vi "12.14.15 Voltage input8inputs.vi"(0 "refnum Write file in":refnum<file>, 1 "Stop in":refnum<vi>, 3 "Number of Samples":i32=100, 4 "Sample Rate":dbl=1000.0, 7 "error in 2":errorcluster, 8 "Display? \nOff/On":bool, 10 "Boolean":bool, 11 "Sample rate (actual)":refnum<vi>, 15 "Plot Output":refnum<vi>, 16 "Plot 1 ref":refnum<vi>, 17 "Plot 2 ref":refnum<vi>) -> (13 "error out 2":errorcluster, 14 "refnum Write file out":refnum<file>, 19 "error out":errorcluster)   [LabVIEW 2017]
uses:
  <vilib>/DAQmx/read.llb/DAQmx Read (Analog 1D Wfm NChan NSamp).vi
  <vilib>/DAQmx/create/channels.llb/DAQmx Create Channel (AI-Voltage-Basic).vi
  <vilib>/DAQmx/configure/timing.llb/DAQmx Timing (Sample Clock).vi
  <vilib>/DAQmx/miscellaneous.llb/DAQmx Fill In Error Info.vi
  <resource>/objmgr/daqmx.rc
panel:
  out "Plot 3":cluster{dbl, dbl, dbl, dbl}(graph)
  out "Plot 1":dbl(graph)
  out "Plot 2":dbl(graph)
  out "Actual Sample Rate":dbl=1000.0 format="%0.2f"
  # "© The Regents of the University of California, Davis campus, 2019. This material is available as open source for research and personal use under a Creative Commons Attribution-NonCommercial-NoDerivatives 4.0 International Public License (https://creativecommons.org/licenses/by-nc-nd/4.0/)."
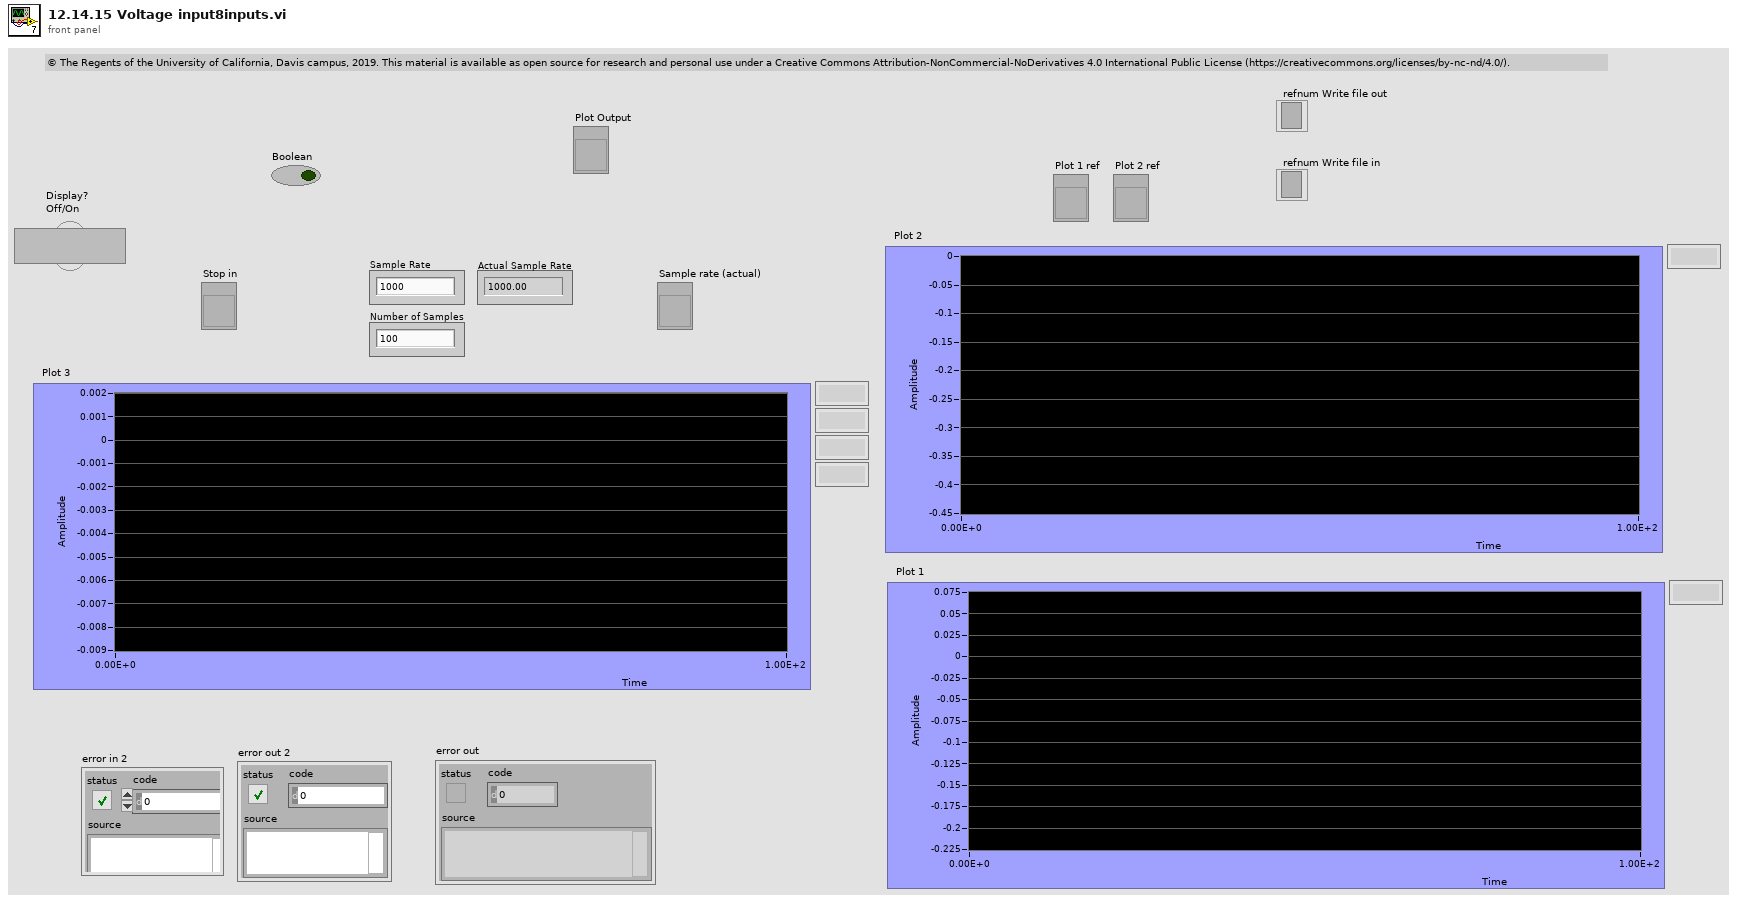
[diagram p1: front panel]
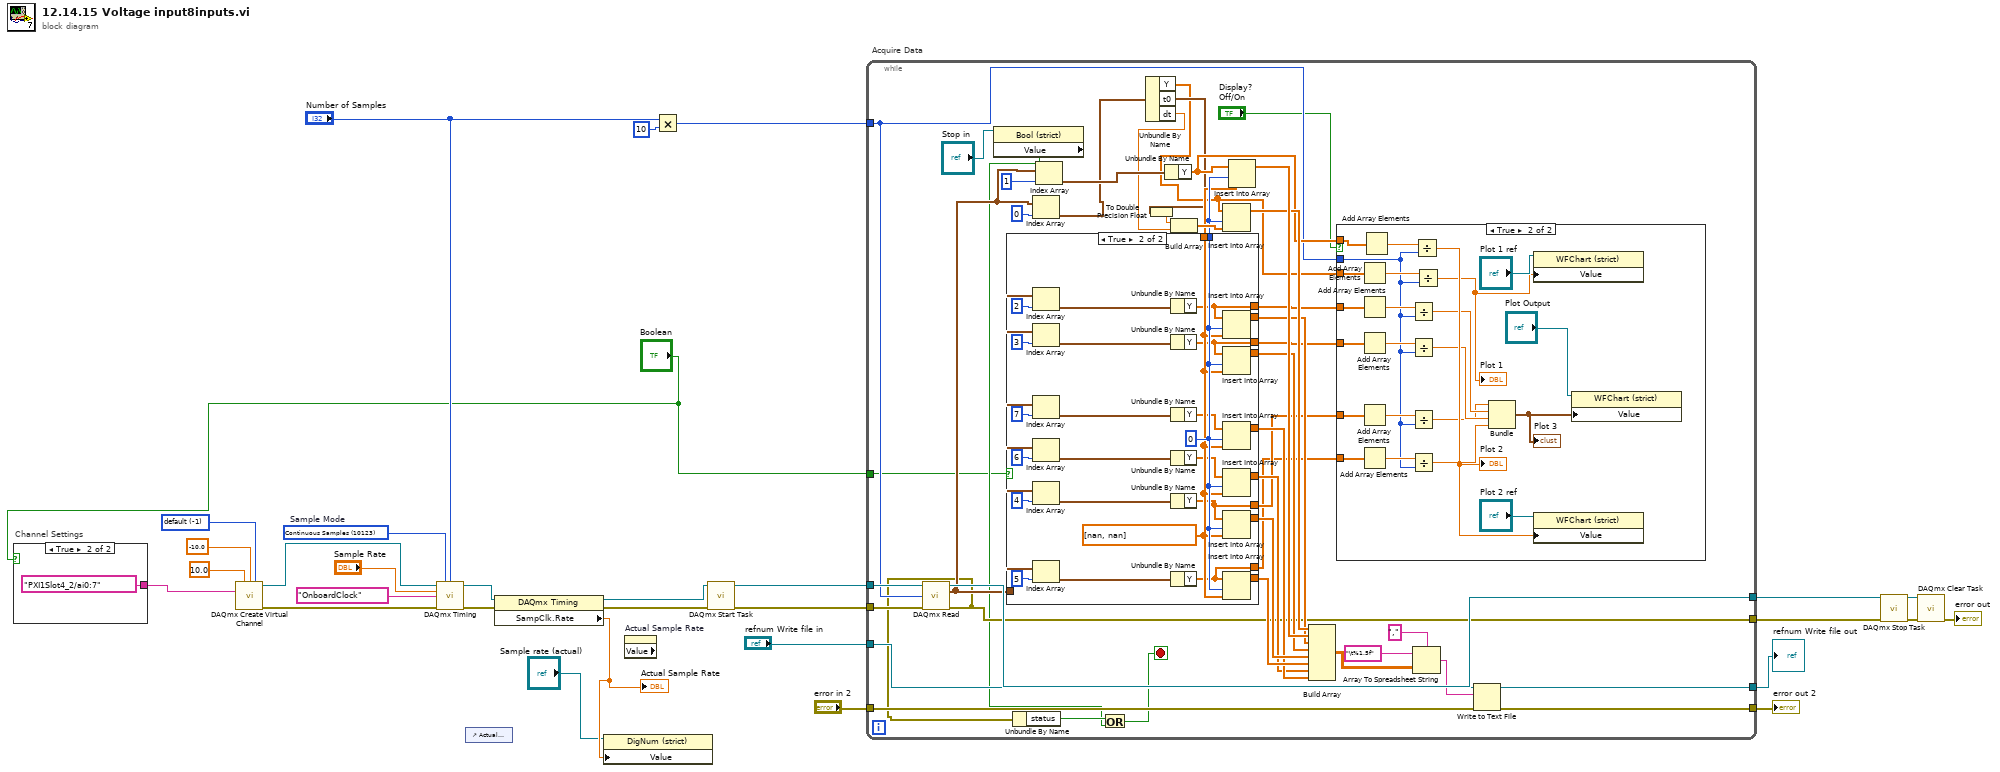
[diagram p0: block diagram]
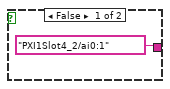
[diagram p2: hidden frame]
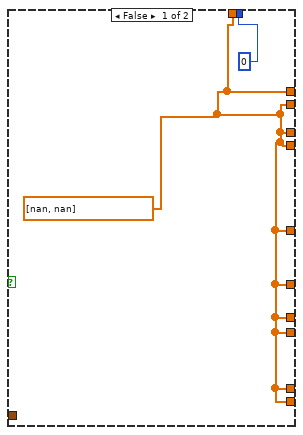
[diagram p3: hidden frame]
diagram:
  w17 = -1 items=["default"=-1, "RSE"=10083, "NRSE"=10078, "Differential"=10106, "Pseudodifferential"=12529] ("Terminal Configuration")
  w20 = 10123 items=["Finite Samples"=10178, "Continuous Samples"=10123, "Hardware Timed Single Point"=12522]  # Sample Mode
  # "Acquire Data"
  # "Channel Settings"
  n1 = case shown="True" "Boolean" {
    tunnel: [tag "PXI1Slot4_2/ai0:1" ("Physical Channel") tag "PXI1Slot4_2/ai0:7" ("Physical Channel")] -> w4
    frame False {
    }
    frame True {
    }
  }
  n2 = call-poly <vilib>:"DAQmx Create Virtual Channel.vi"("maximum value"=10.0 ("Min Voltage"), "minimum value"=-10.0 ("Min Voltage"), "input terminal configuration"=w17, "physical channels"=w4) -> ("task out"=w27:refnum<k21>, "error out"=w28:errorcluster)  [unwired: 10 in]
  n3 = call-poly <vilib>:"DAQmx Timing.vi"("task/channels in"=w27, "sample mode"=w20, "samples per channel"="Number of Samples", "rate"="Sample Rate", "source"=tag "OnboardClock" ("Sample Clock Source"), "error in"=w28) -> ("task out"=w30:refnum<k21>, "error out"=w29:errorcluster)  [unwired: 8 in]
  n4 = control-ref of="Actual Sample Rate"() -> ()  [unwired: 1 out]
  n5 = property class="DAQmx Timing"(reference=w30, error in=w29) -> (reference out=w12:refnum<k21>, error out=w11:errorcluster, "SampClk.Rate"=w2:dbl)
  "Actual Sample Rate" <- w2
  n6 = property on="Property Node" class="DigNum (strict)"(reference="Sample rate (actual)", "Value"=w2) -> ()  [unwired: 1 in, 2 out]
  n7 = property on="Actual Sample Rate" class="DigNum (strict)" props=["Value"]() -> ()  [unwired: 2 in, 3 out]
  n8 = Multiply(x="Number of Samples", y=10 ("Number of Samples")) -> (x*y=w5:i32)
  n9 = call <vilib>:"DAQmx Start Task.vi"("task/channels in"=w12, "error in"=w11) -> ("task out"=w26:refnum<k21>, "error out"=w15:errorcluster)  [unwired: 12 in]
  n10 = while {
    tunnel: w26 -> [w76]
    tunnel: [w75] -> w24
    tunnel: w5 -> [w45]
    tunnel: w15 -> [w74]
    tunnel: [w36] -> w14
    tunnel: [w71] -> w13
    tunnel: "error in 2" -> [w68]
    tunnel: [w67] -> w9
    tunnel: "refnum Write file in" -> [w66]
    tunnel: "Boolean" -> [w33]
    stop <- w35 stop-if-true
    n11 = call-poly <vilib>:"DAQmx Read.vi"("task/channels in"=w76, "number of samples per channel"=w45, "error in"=w74) -> ("task out"=w75:refnum<k21>, "data"=w58:waveform(dbl)[], "error out"=w36:errorcluster)  [unwired: 10 in]
    n12 = property on="Property Node" class="Bool (strict)"(reference="Stop in") -> ("Value"=w34:bool)  [unwired: 1 in, 2 out]
    n13 = case shown="True" w33 {
      tunnel: w58 -> [_ w93]
      tunnel: [w78 w92] -> w57
      tunnel: [w78 w91] -> w56
      tunnel: [w78 w90] -> w55
      tunnel: [w78 w89] -> w54
      tunnel: [0 ("index (row)") w88] -> w53
      tunnel: [w78 w87] -> w52
      tunnel: [w78 w86] -> w49
      tunnel: [w78 w85] -> w48
      tunnel: [w78 w84] -> w47
      tunnel: [w78 w82] -> w46
      tunnel: [w78 w80] -> w43
      tunnel: [w78 w79] -> w42
      frame False {
        w78 = dbl[] [nan, nan] ("new element/subarray")
      }
      frame True {
        w87 = dbl[] [nan, nan] ("new element/subarray")
        w88 = 0 ("index (row)")
        n14 = Index Array(array=w93, index=2) -> (element=w105:waveform(dbl))
        n15 = Index Array(array=w93, index=3) -> (element=w102:waveform(dbl))
        n16 = Index Array(array=w93, index=7) -> (element=w94:waveform(dbl))
        n17 = Index Array(array=w93, index=6) -> (element=w97:waveform(dbl))
        n18 = Index Array(array=w93, index=4) -> (element=w101:waveform(dbl))
        n19 = Index Array(array=w93, index=5) -> (element=w98:waveform(dbl))
        n20 = Unbundle By Name(w105) -> ("Y"=w82:dbl[])
        n21 = Unbundle By Name(w102) -> ("Y"=w84:dbl[])
        n22 = Unbundle By Name(w94) -> ("Y"=w81:dbl[])
        n23 = Unbundle By Name(w97) -> ("Y"=w83:dbl[])
        n24 = Unbundle By Name(w101) -> ("Y"=w80:dbl[])
        n25 = Unbundle By Name(w98) -> ("Y"=w79:dbl[])
        n26 = Insert Into Array(array=w82, index=w88, new element=w87) -> (w92:dbl[])
        n27 = Insert Into Array(array=w84, index=w88, new element=w87) -> (w86:dbl[])
        n28 = Insert Into Array(array=w81, index=w88, new element=w87) -> (w89:dbl[])
        n29 = Insert Into Array(array=w83, index=w88, new element=w87) -> (w85:dbl[])
        n30 = Insert Into Array(array=w80, index=w88, new element=w87) -> (w91:dbl[])
        n31 = Insert Into Array(array=w79, index=w88, new element=w87) -> (w90:dbl[])
      }
    }
    n32 = Unbundle By Name(w36) -> ("status"=w37:bool)
    n33 = Index Array(array=w58, index=0 ("index (row)")) -> (element=w41:waveform(dbl))
    n34 = Index Array(array=w58, index=1) -> (element=w64:waveform(dbl))
    n35 = Or(x=w37, y=w34) -> (x .or. y?=w35:bool)
    n36 = Unbundle By Name(w41) -> ("Y"=w38:dbl[], "t0"=w39:timestamp, "dt"=w40:dbl)
    n37 = To Double Precision Float(number=w39) -> (double precision float=w63:dbl)
    n38 = Unbundle By Name(w64) -> ("Y"=w51:dbl[])
    n39 = Build Array(w63, w40) -> (w62:dbl[])
    n40 = Insert Into Array(array=w38, index=w53, new element=w62) -> (w60:dbl[])
    n41 = Insert Into Array(array=w51, index=w53, new element=w52) -> (w61:dbl[])
    n42 = Build Array(w60, w61, w57, w49, w56, w55, w48, w54) -> (w59:dbl[][])
    n43 = case shown="True" "Display? \nOff/On" {
      tunnel: w38 -> [_ w126]
      tunnel: w51 -> [_ w125]
      tunnel: w47 -> [_ w118]
      tunnel: w42 -> [_ w117]
      tunnel: w46 -> [_ w113]
      tunnel: w45 -> [_ w110]
      tunnel: w43 -> [_ w109]
      frame False {
      }
      frame True {
        n44 = Add Array Elements(numeric array=w126) -> (sum=w128:dbl)
        n45 = Add Array Elements(numeric array=w113) -> (sum=w115:dbl)
        n46 = Add Array Elements(numeric array=w118) -> (sum=w120:dbl)
        n47 = Add Array Elements(numeric array=w109) -> (sum=w112:dbl)
        n48 = Add Array Elements(numeric array=w117) -> (sum=w119:dbl)
        n49 = Add Array Elements(numeric array=w125) -> (sum=w127:dbl)
        n50 = Divide(x=w115, y=w110) -> (x/y=w114:dbl)
        n51 = Divide(x=w120, y=w110) -> (x/y=w116:dbl)
        n52 = Divide(x=w112, y=w110) -> (x/y=w111:dbl)
        n53 = Divide(x=w119, y=w110) -> (x/y=w108:dbl)
        n54 = Divide(x=w127, y=w110) -> (x/y=w124:dbl)
        "Plot 2" <- w124
        n55 = Divide(x=w128, y=w110) -> (x/y=w121:dbl)
        "Plot 1" <- w121
        n56 = Bundle(w111, w114, w116, w108) -> (w107:cluster{dbl, dbl, dbl, dbl})  [unwired: 1 in]
        "Plot 3" <- w107
        n57 = property on="Property Node" class="WFChart (strict)"(reference="Plot 1 ref", "Value"=w121) -> ()  [unwired: 1 in, 2 out]
        n58 = property on="Property Node" class="WFChart (strict)"(reference="Plot 2 ref", "Value"=w124) -> ()  [unwired: 1 in, 2 out]
        n59 = property on="Property Node" class="WFChart (strict)"(reference="Plot Output", "Value"=w107) -> ()  [unwired: 1 in, 2 out]
      }
    }
    n60 = Array To Spreadsheet String(delimiter (Tab)=",", array=w59, 3:"\t%1.5f" ("format string")) -> (spreadsheet string=w70:string)
    n61 = Write to Text File(file (use dialog)=w66, text=w70, error in=w68) -> (refnum out=w71:refnum<file>, error out=w67:errorcluster)  [unwired: 1 in, 1 out]
  }
  "refnum Write file out" <- w13
  "error out 2" <- w9
  n62 = call <vilib>:"DAQmx Stop Task.vi"("task/channels in"=w24, "error in"=w14) -> ("task out"=w22:refnum<k21>, "error out"=w23:errorcluster)  [unwired: 12 in]
  n63 = call <vilib>:"DAQmx Clear Task.vi"("task in"=w22, "error in"=w23) -> ("error out"=→"error out":errorcluster)  [unwired: 13 in]
